vi "GenerateCode.vi"(1 "Terms":T13[](array[typedef]), 3 "Diagram":refnum<vi>, 5 "XRef":refnum<vi>, 6 "State In":T1) -> (0 "Generated Code?":bool, 2 "State Out":T1, 4 "Reply":string[](array[string]))   [LabVIEW 2017]
uses:
  <vilib>/XNodeSupport/XNodeTermIDPair.ctl
  <vilib>/XNodeSupport/XNodeTermRef.ctl
  <vilib>/XNodeSupport/XNodeString.ctl
  <vilib>/UPVI/lvhdf5/xnodehelpers/State.ctl
  <vilib>/UPVI/lvhdf5/xnodehelpers/TermsPlus.ctl
  <vilib>/XNodeSupport/XNodeTerm3.ctl
  <vilib>/XNodeSupport/XNodeVariant.ctl
  <vilib>/XNodeSupport/XNodeRect32.ctl
  <vilib>/XNodeSupport/XNodeInt.ctl
  <vilib>/XNodeSupport/XNodeBool.ctl
  <vilib>/XNodeSupport/XNodeTermDirection.ctl
  <vilib>/UPVI/lvhdf5/xnodehelpers/TermBehavior.ctl
  <vilib>/XNodeSupport/XNodeError3Array.ctl
  <vilib>/XNodeSupport/XNodeError3.ctl
  <vilib>/Utility/traverseref.llb/TRef TravTarget.ctl
  <vilib>/Utility/VariantDataType/Type.ctl
  <vilib>/Utility/traverseref.llb/VI Scripting - Traverse.lvlib
  <vilib>/Utility/VariantDataType/VariantType.lvlib
  <vilib>/XNodeSupport/NI_XNodeSupport.lvlib
panel:
  in  "vi path":path
  # "LVHDF5 Toolkit\nCopyright (c) 2005-2013 by Jason D. Sommerville\nCopyright (c) 2014 by UPVI, LLC.\n\nThis use and distribution of this file is governed by the terms found in \nLICENSE.txt distributed with this toolkit and installed at\n <user.lib>\\_lvhdf5\\LICENSE.txt"
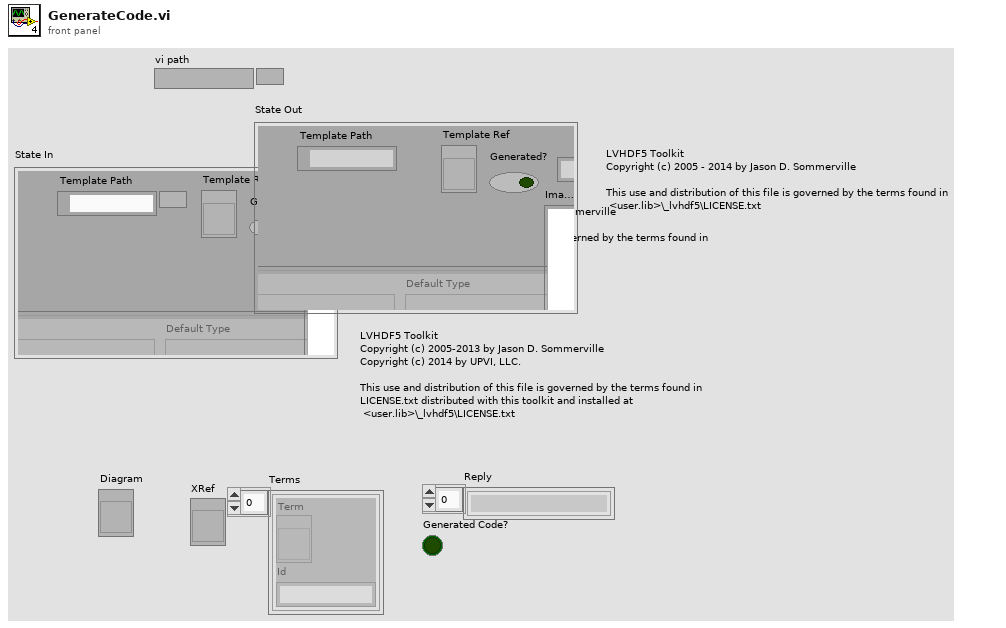
[diagram p1: front panel]
types:
  T1 = typedef "State.ctl" = cluster{"Template Path":path, "Template Ref":refnum<vi>, "Terms":T2[], "Display Name":string, "Image":picture, "Errors":T11, "Generated?":bool}
  T2 = typedef "TermsPlus.ctl" = cluster{"Term 3":T3, "Default Type":variant, "Behavior":T10, "Behavior Arg":string, "WiredResponse":bool, "Wired":enum16{"Unknown", "Unwired", "Wired"}}
  T3 = typedef "NI_XNodeSupport.lvlib/XNodeTerm3.ctl" = cluster{"Name":T4, "Id":T4, "Type":T5, "Bounds":T6, "Input?":T8, "Required?":T8, "Recommended?":T8, "Adaptive?":T8, "Hidden?":T8, "Direction":T9, "Break Wire?":T8}
  T4 = typedef "NI_XNodeSupport.lvlib/XNodeString.ctl" = string
  T5 = typedef "NI_XNodeSupport.lvlib/XNodeVariant.ctl" = variant
  T6 = typedef "NI_XNodeSupport.lvlib/XNodeRect32.ctl" = cluster{"Left":T7, "Top":T7, "Right":T7, "Bottom":T7}
  T7 = typedef "NI_XNodeSupport.lvlib/XNodeInt.ctl" = i32
  T8 = typedef "NI_XNodeSupport.lvlib/XNodeBool.ctl" = bool
  T9 = typedef "NI_XNodeSupport.lvlib/XNodeTermDirection.ctl" = enum32{"Auto", "Up", "Down", "Left", "Right", "Center"}
  T10 = typedef "TermBehavior.ctl" = enum16{"Normal", "Anything", "LVType", "Path or Ref", "Attr Name", "Attr Poly", "Elt Poly", "Dset Poly", "WDT Poly"}
  T11 = typedef "NI_XNodeSupport.lvlib/XNodeError3Array.ctl" = T12[]
  T12 = typedef "NI_XNodeSupport.lvlib/XNodeError3.ctl" = cluster{"Error":T4, "Details":T4, "Help File":T4, "Help Topic":T4}
  T13 = typedef "NI_XNodeSupport.lvlib/XNodeTermIDPair.ctl" = cluster{"Term":T14, "Id":T4}
  T14 = typedef "NI_XNodeSupport.lvlib/XNodeTermRef.ctl" = refnum<vi>
  T15 = typedef "TRef TravTarget.ctl" = enum16{"FP", "BD", "Other"}
  T16 = typedef "VariantType.lvlib/Type.ctl" = enum8{"Invalid Type", "Void", "I8", "I16", "I32", "I64", "U8", "U16", "U32", "U64", "Single Float", "Double Float", "Extended Float", "Single Complex", "Double Complex", "Extended Complex", "Enum U8", "Enum U16", "Enum U32", "Enum U64", "Single Float With Unit", "Double Float With Unit", "Extended Float With Unit", "Single Complex with Unit", "Double Complex with Unit", "Extended Complex with Unit", "Boolean", "String", "Path", "Picture", "Tag", "Array", "Cluster", "Variant", "LV Variant", "Waveform", "Timestamp", "Digital Waveform", "Digital Data", "ExpressData", "Refnum", "External Data", "VI", "Poly VI", "LabVIEW Class Instance", "Fixed Point"}
  T17 = typedef "LVPositionTypeDef.ctl" = cluster{"Left":i32, "Top":i32}
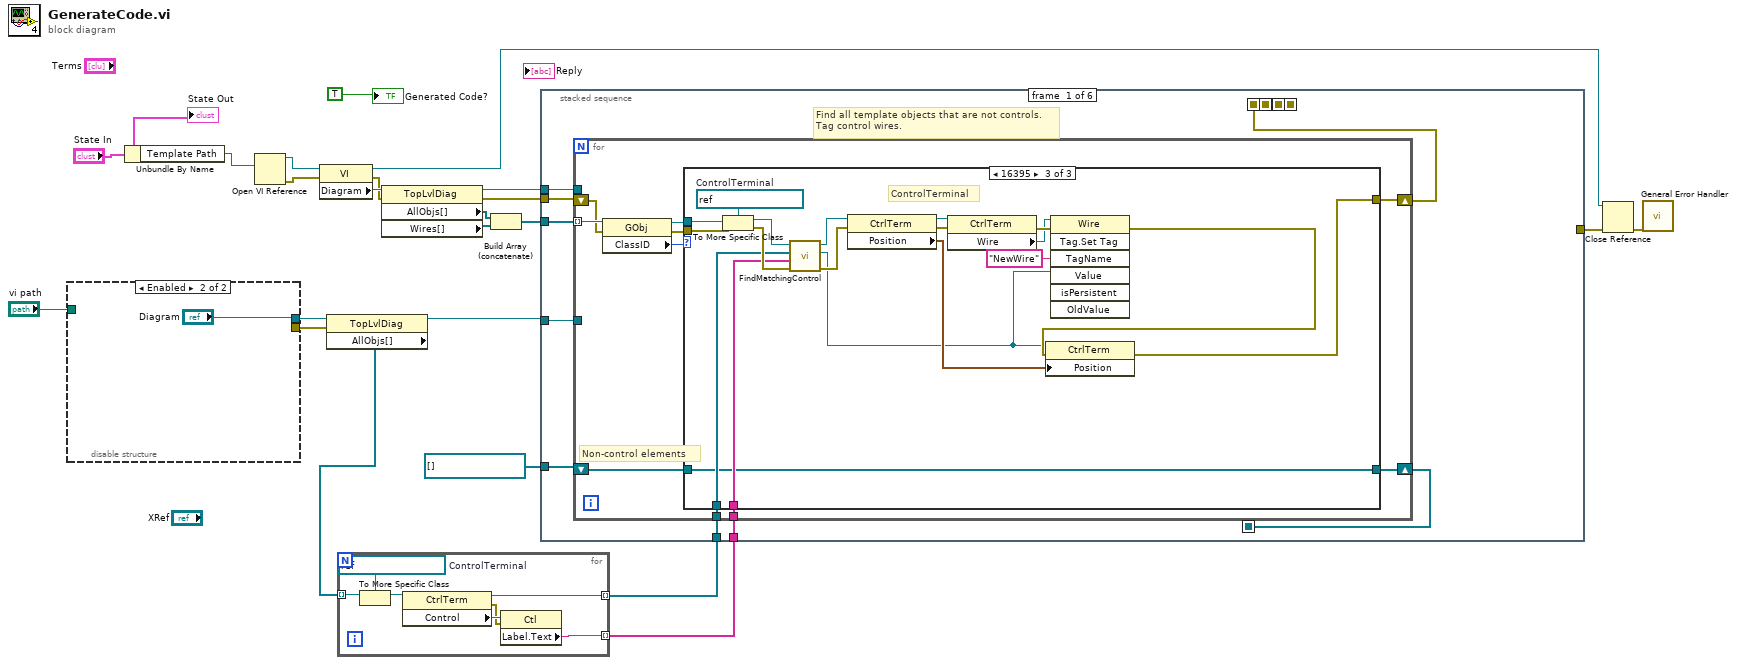
[diagram p0: block diagram]
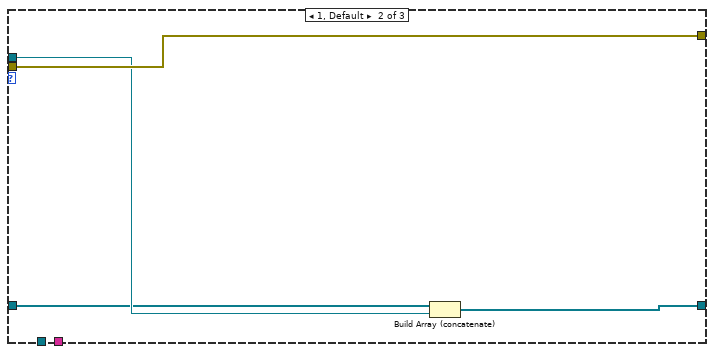
[diagram p3: hidden frame]
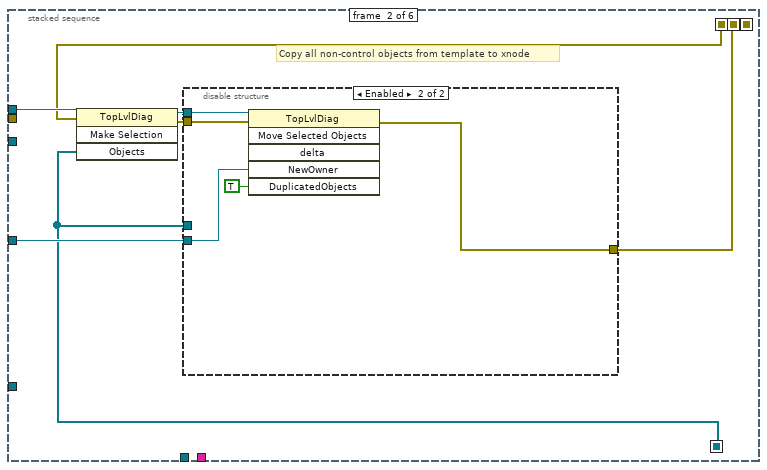
[diagram p4: hidden frame]
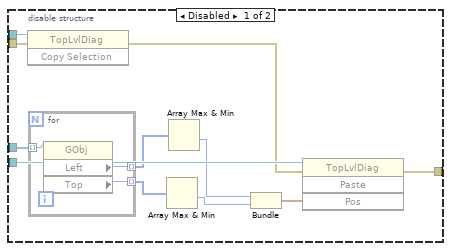
[diagram p5: hidden frame]
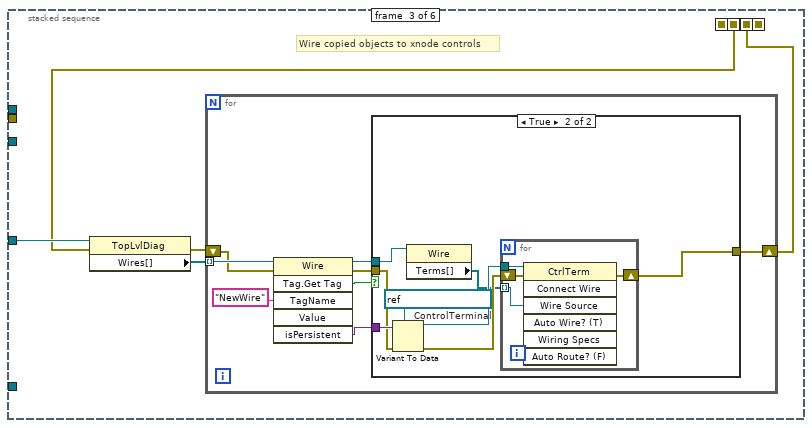
[diagram p6: hidden frame]
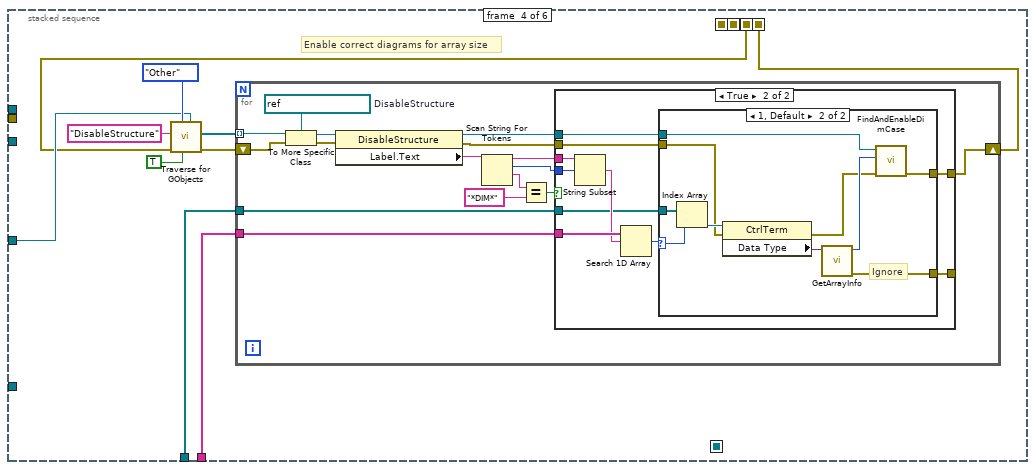
[diagram p8: hidden frame]
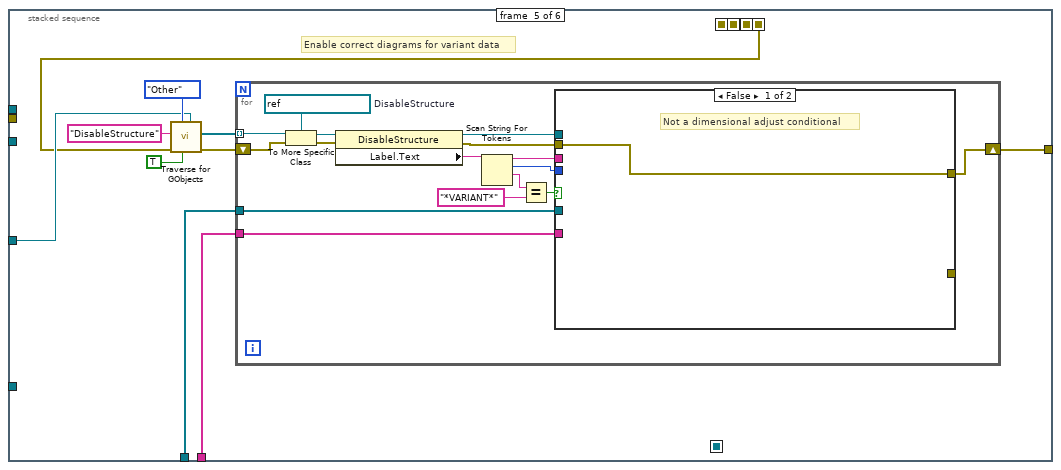
[diagram p11: hidden frame]
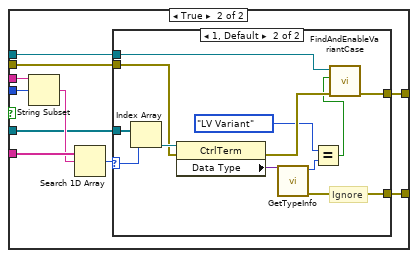
[diagram p12: hidden frame]
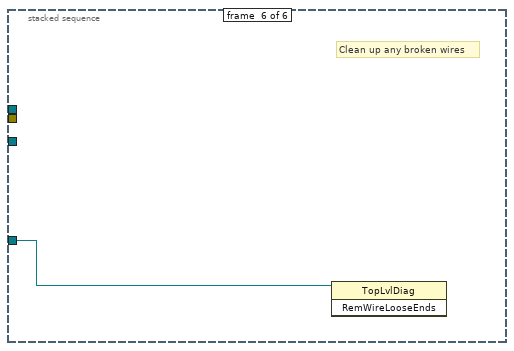
[diagram p14: hidden frame]
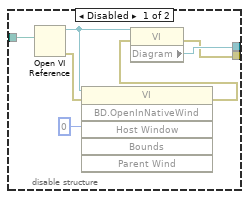
[diagram p15: hidden frame]
diagram:
  n1 = disable-structure shown="Enabled" {
    disable-tunnel: "vi path" -> [w30 _]
    disable-tunnel: [w29 "Diagram"] -> w19
    disable-tunnel: [w28 _] -> w7
    frame Disabled {
      n2 = Open VI Reference(vi path=w30) -> (vi reference=w27:refnum<vi>, error out=w26:errorcluster)  [unwired: 5 in]
      n3 = invoke class="VI" method="BD.OpenInNativeWind"(reference=w27, error in=w26, "Host Window"=u64 0) -> (error out=w25:errorcluster)  [unwired: 3 in, 5 out]
      n4 = property class="VI"(reference=w27, error in=w25) -> (error out=w28:errorcluster, "Diagram"=w29:refnum<vi>)  [unwired: 1 out]
    }
    frame Enabled {
    }
  }
  n5 = Unbundle By Name("State In") -> ("Template Path"=w6:path)
  n6 = Open VI Reference(vi path=w6) -> (vi reference=w4:refnum<vi>, error out=w5:errorcluster)  [unwired: 5 in]
  n7 = property class="VI"(reference=w4, error in=w5) -> (reference out=w1:refnum<vi>, error out=w20:errorcluster, "Diagram"=w23:refnum<vi>)
  n8 = property class="TopLvlDiag"(reference=w19, error in=w7) -> (reference out=w9:refnum<vi>, "AllObjs[]"=w18:refnum<vi>[])  [unwired: 1 out]
  n9 = for {
    tunnel: w18 -> [w38] mode=indexing
    tunnel: [w33] -> w10 mode=indexing
    tunnel: [w32] -> w11 mode=indexing
    w37 = refnum<vi> refnum  # ControlTerminal
    n10 = To More Specific Class(target class=w37, reference=w38) -> (specific class reference=w36:refnum<vi>)  [unwired: 1 in, 1 out]
    n11 = property class="CtrlTerm"(reference=w36) -> (reference out=w32:refnum<vi>, error out=w34:errorcluster, "Control"=w35:refnum<vi>)  [unwired: 1 in]
    n12 = property class="Ctl"(reference=w35, error in=w34) -> ("Label.Text"=w33:string)  [unwired: 2 out]
  }
  n13 = property class="TopLvlDiag"(reference=w23, error in=w20) -> (reference out=w14:refnum<vi>, error out=w13:errorcluster, "AllObjs[]"=w21:refnum<vi>[], "Wires[]"=w17:refnum<vi>[])
  n14 = Build Array (concatenate)(w21, w17) -> (w12:refnum<vi>[])
  n15 = stacked-sequence {
    seq-local: [w40 _ _ _ _ _] -> [_ w83 _ _ _ _]
    seq-local: [w43 _ _ _ _ _] -> [_ w85 _ _ _ _]
    seq-local: [_ w84 _ _ _ _] -> [_ _ w109 _ _ _]
    seq-local: [_ _ w110 _ _ _] -> [_ _ _ w139 _ _]
    seq-local: [_ _ _ w135 _ _] -> [_ _ _ _ w184 _]
    tunnel: w12 -> [w47 _ _ _ _ _]
    tunnel: w14 -> [w46 w89 _ _ _ _]
    tunnel: w13 -> [w41 _ _ _ _ _]
    tunnel: w10 -> [w45 _ _ w137 w186 _]
    tunnel: w9 -> [w44 w86 w111 w141 w189 w233]
    tunnel: w11 -> [w42 _ _ w136 w185 _]
    tunnel: [_ _ _ _ w183 _] -> w3
    tunnel: refnum<vi>[] [] -> [w39 _ _ _ _ _]
    frame #0 {
      # "Find all template objects that are not controls.\nTag control wires."
      n16 = for {
        tunnel: w47 -> [w57] mode=indexing
        tunnel: w46 -> [_]
        shift-right: [w50] -> w43
        shift-left: w41 -> [w56]
        tunnel: w45 -> [w51]
        tunnel: w44 -> [_]
        tunnel: w42 -> [w52]
        shift-right: [w49] -> w40
        shift-left: w39 -> [w48]
        # "Non-control elements"
        n17 = property class="GObj"(reference=w57, error in=w56) -> (reference out=w53:refnum<vi>, error out=w54:errorcluster, "ClassID"=w55:u32)
        n18 = case shown="16395" w55 {
          tunnel: w53 -> [_ w62 w81]
          tunnel: w54 -> [w59 w63 w80]
          tunnel: w51 -> [_ _ w65]
          tunnel: [w59 w63 w74] -> w50
          tunnel: w52 -> [_ _ w66]
          tunnel: [w58 w61 w64] -> w49
          tunnel: w48 -> [w58 w60 w64]
          frame 0 {
          }
          frame 1, Default {
            n19 = Build Array (concatenate)(w60, w62) -> (w61:refnum<vi>[])
          }
          frame 16395 {
            w82 = refnum<vi> refnum  # ControlTerminal
            # "ControlTerminal"
            n20 = To More Specific Class(target class=w82, reference=w81, error in=w80) -> (specific class reference=w78:refnum<vi>, error out=w79:errorcluster)
            n21 = call <vilib>:"FindMatchingControl.vi"("error in"=w79, "ControlNames"=w65, "ControlIDs"=w66, "Source Ctrl Ref"=w78) -> ("error out"=w75:errorcluster, "Target Ctrl Ref"=w68:refnum<vi>, "Source Ctrl Ref out"=w77:refnum<vi>)  [unwired: 1 in, 2 out]
            n22 = property class="CtrlTerm"(reference=w77, error in=w75) -> (reference out=w73:refnum<vi>, error out=w72:errorcluster, "Position"=w76:T17)
            n23 = property class="CtrlTerm"(reference=w73, error in=w72) -> (error out=w71:errorcluster, "Wire"=w67:refnum<vi>)  [unwired: 1 out]
            n24 = invoke class="Wire" method="Tag.Set Tag"(reference=w67, error in=w71, "TagName"="NewWire" ("Tag Name"), "Value"=w68) -> (error out=w69:errorcluster)  [unwired: 3 in, 6 out]
            n25 = property class="CtrlTerm"(reference=w68, error in=w69, "Position"=w76) -> (error out=w74:errorcluster)  [unwired: 1 out]
          }
        }
      }
    }
    frame #1 {
      # "Copy all non-control objects from template to xnode"
      n26 = invoke class="TopLvlDiag" method="Make Selection"(reference=w89, error in=w85, "Objects"=w83) -> (reference out=w88:refnum<vi>, error out=w87:errorcluster)  [unwired: 1 in, 2 out]
      n27 = disable-structure shown="Enabled" {
        disable-tunnel: w88 -> [w100 w108]
        disable-tunnel: w87 -> [w99 w107]
        disable-tunnel: w86 -> [w98 w106]
        disable-tunnel: [w96 w104] -> w84
        disable-tunnel: w83 -> [w90 _]
        frame Disabled {
          n28 = invoke class="TopLvlDiag" method="Copy Selection"(reference=w100, error in=w99) -> (error out=w97:errorcluster)  [unwired: 1 in, 2 out]
          n29 = for {
            tunnel: w90 -> [w103] mode=indexing
            tunnel: [w102] -> w94 mode=indexing
            tunnel: [w101] -> w95 mode=indexing
            n30 = property class="GObj"(reference=w103) -> ("Left"=w102:i32, "Top"=w101:i32)  [unwired: 1 in, 2 out]
          }
          n31 = Array Max & Min(array=w95) -> (min value=w92:i32)  [unwired: 3 out]
          n32 = Array Max & Min(array=w94) -> (min value=w93:i32)  [unwired: 3 out]
          n33 = Bundle(w93, w92) -> (w91:cluster{i32, i32})  [unwired: 1 in]
          n34 = invoke class="TopLvlDiag" method="Paste"(reference=w98, error in=w97, "Pos"=w91) -> (error out=w96:errorcluster)  [unwired: 1 in, 3 out]
        }
        frame Enabled {
          n35 = invoke class="TopLvlDiag" method="Move Selected Objects"(reference=w108, error in=w107, "NewOwner"=w106, "DuplicatedObjects"=TRUE ("Duplicate?")) -> (error out=w104:errorcluster)  [unwired: 2 in, 5 out]
        }
      }
    }
    frame #2 {
      # "Wire copied objects to xnode controls"
      n36 = property class="TopLvlDiag"(reference=w111, error in=w109) -> (error out=w112:errorcluster, "Wires[]"=w113:refnum<vi>[])  [unwired: 1 out]
      n37 = for {
        tunnel: w113 -> [w121] mode=indexing
        shift-right: [w114] -> w110
        shift-left: w112 -> [w117]
        n38 = invoke class="Wire" method="Tag.Get Tag"(reference=w121, error in=w117, "TagName"="NewWire" ("Tag Name")) -> (reference out=w115:refnum<vi>, error out=w116:errorcluster, "GetTag"=w118:bool, "isPersistent"=w119:variant)  [unwired: 3 in, 2 out]
        n39 = case shown="True" w118 {
          tunnel: w119 -> [_ w130]
          tunnel: w116 -> [w122 w129]
          tunnel: w115 -> [_ w124]
          tunnel: [w122 w125] -> w114
          frame False {
          }
          frame True {
            w128 = refnum<vi> refnum  # ControlTerminal
            n40 = Variant To Data(error in=w129, type=w128, Variant=w130) -> (data=w127:refnum<vi>, error out=w126:errorcluster)
            n41 = property class="Wire"(reference=w124) -> ("Terms[]"=w123:refnum<vi>[])  [unwired: 1 in, 2 out]
            n42 = for {
              tunnel: w127 -> [w134]
              shift-right: [w132] -> w125
              shift-left: w126 -> [w133]
              tunnel: w123 -> [w131] mode=indexing
              n43 = invoke class="CtrlTerm" method="Connect Wire"(reference=w134, error in=w133, "Wire Source"=w131) -> (error out=w132:errorcluster)  [unwired: 4 in, 6 out]
            }
          }
        }
      }
    }
    frame #3 {
      # "Enable correct diagrams for array size"
      n44 = call <vilib>:"Traverse for GObjects.vi"("Other Refnum"=w141, "Traverse Generated Code (F)"=TRUE, "Traverse Target"=TRef_TravTarget."Other", "error in (no error)"=w139, "Class Name"="DisableStructure") -> ("error out"=w138:errorcluster, "References"=w140:refnum<vi>[])  [unwired: 3 in, 2 out]
      n45 = for {
        tunnel: w140 -> [w160] mode=indexing
        shift-right: [w145] -> w135
        shift-left: w138 -> [w158]
        tunnel: w137 -> [w149]
        tunnel: w136 -> [w148]
        w159 = refnum<vi> refnum  # DisableStructure
        n46 = To More Specific Class(target class=w159, reference=w160, error in=w158) -> (specific class reference=w157:refnum<vi>, error out=w156:errorcluster)
        n47 = property class="DisableStructure"(reference=w157, error in=w156) -> (reference out=w147:refnum<vi>, error out=w146:errorcluster, "Label.Text"=w155:string)
        n48 = Scan String For Tokens(9:w155) -> (1:w154:string, 2:w150:i32, 3:w151:string)  [unwired: 5 in, 1 out]
        n49 = Equal?(x=w154, y="*DIM*") -> (x = y?=w152:bool)
        n50 = case shown="True" w152 {
          tunnel: w151 -> [_ w171]
          tunnel: w150 -> [_ w170]
          tunnel: w149 -> [_ w169]
          tunnel: w148 -> [_ w167]
          tunnel: w147 -> [_ w165]
          tunnel: w146 -> [w161 w164]
          tunnel: [w161 w163] -> w145
          tunnel: [_ w162] -> _
          frame False {
            # "Not a dimensional adjust conditional"
          }
          frame True {
            n51 = String Subset(string=w171, offset (0)=w170) -> (substring=w168:string)  [unwired: 1 in]
            n52 = Search 1D Array(1D array=w169, element=w168) -> (index of element=w166:i32)  [unwired: 1 in]
            n53 = case shown="1, Default" w166 {
              selector: w166 -> [_ w181]
              tunnel: w167 -> [_ w182]
              tunnel: w165 -> [_ w178]
              tunnel: w164 -> [w172 w176]
              tunnel: [w172 w174] -> w163
              tunnel: [_ w173] -> w162
              frame -1 {
                # "Control not found\nDo nothing"
              }
              frame 1, Default {
                # "Ignore"
                n54 = Index Array(array=w182, index=w181) -> (element=w180:refnum<vi>)
                n55 = property class="CtrlTerm"(reference=w180, error in=w176) -> (error out=w175:errorcluster, "Data Type"=w179:variant)  [unwired: 1 out]
                n56 = call <vilib>:"GetArrayInfo.vi"("Variant"=w179) -> ("error out"=w173:errorcluster, "NDims"=w177:i32)  [unwired: 7 in, 2 out]
                n57 = call <vilib>:"FindAndEnableDimCase.vi"("error in (no error)"=w175, "Rank"=w177, "DisableStructure ref"=w178) -> ("error out"=w174:errorcluster)  [unwired: 5 in, 3 out]
              }
            }
          }
        }
      }
    }
    frame #4 {
      # "Enable correct diagrams for variant data"
      n58 = call <vilib>:"Traverse for GObjects.vi"("Other Refnum"=w189, "Traverse Generated Code (F)"=TRUE, "Traverse Target"=TRef_TravTarget."Other", "error in (no error)"=w184, "Class Name"="DisableStructure") -> ("error out"=w187:errorcluster, "References"=w188:refnum<vi>[])  [unwired: 3 in, 2 out]
      n59 = for {
        tunnel: w188 -> [w208] mode=indexing
        shift-right: [w193] -> w183
        shift-left: w187 -> [w206]
        tunnel: w186 -> [w197]
        tunnel: w185 -> [w196]
        w207 = refnum<vi> refnum  # DisableStructure
        n60 = To More Specific Class(target class=w207, reference=w208, error in=w206) -> (specific class reference=w205:refnum<vi>, error out=w204:errorcluster)
        n61 = property class="DisableStructure"(reference=w205, error in=w204) -> (reference out=w195:refnum<vi>, error out=w194:errorcluster, "Label.Text"=w203:string)
        n62 = Scan String For Tokens(9:w203) -> (1:w202:string, 2:w198:i32, 3:w199:string)  [unwired: 5 in, 1 out]
        n63 = Equal?(x=w202, y="*VARIANT*") -> (x = y?=w200:bool)
        n64 = case shown="False" w200 {
          tunnel: w199 -> [_ w219]
          tunnel: w198 -> [_ w218]
          tunnel: w197 -> [_ w217]
          tunnel: w196 -> [_ w215]
          tunnel: w195 -> [_ w213]
          tunnel: w194 -> [w209 w212]
          tunnel: [w209 w211] -> w193
          tunnel: [_ w210] -> _
          frame False {
            # "Not a dimensional adjust conditional"
          }
          frame True {
            n65 = String Subset(string=w219, offset (0)=w218) -> (substring=w216:string)  [unwired: 1 in]
            n66 = Search 1D Array(1D array=w217, element=w216) -> (index of element=w214:i32)  [unwired: 1 in]
            n67 = case shown="1, Default" w214 {
              selector: w214 -> [_ w231]
              tunnel: w215 -> [_ w232]
              tunnel: w213 -> [_ w229]
              tunnel: w212 -> [w220 w228]
              tunnel: [w220 w226] -> w211
              tunnel: [_ w224] -> w210
              frame -1 {
                # "Control not found\nDo nothing"
              }
              frame 1, Default {
                # "Ignore"
                n68 = Index Array(array=w232, index=w231) -> (element=w230:refnum<vi>)
                n69 = property class="CtrlTerm"(reference=w230, error in=w228) -> (error out=w227:errorcluster, "Data Type"=w225:variant)  [unwired: 1 out]
                n70 = call <vilib>:"GetTypeInfo.vi"("Variant"=w225) -> ("error out"=w224:errorcluster, "Type Enum"=w223:T16)  [unwired: 6 in, 3 out]
                n71 = Equal?(x=Type."LV Variant" ("Type Enum"), y=w223) -> (x = y?=w221:bool)
                n72 = call <vilib>:"FindAndEnableVariantCase.vi"("error in (no error)"=w227, "Control Is Variant"=w221, "DisableStructure ref"=w229) -> ("error out"=w226:errorcluster)  [unwired: 5 in, 3 out]
              }
            }
          }
        }
      }
    }
    frame #5 {
      # "Clean up any broken wires"
      n73 = invoke class="TopLvlDiag" method="RemWireLooseEnds"(reference=w233) -> ()  [unwired: 2 in, 3 out]
    }
  }
  n74 = Close Reference(reference=w1, error in (no error)=w3) -> (error out=w2:errorcluster)
  n75 = call <vilib>:"General Error Handler.vi"("error in (no error)"=w2) -> ()  [unwired: 10 in, 5 out]
  "Generated Code?" <- TRUE ("Generated Code?")
  "State Out" <- "State In"
